vi "Build FilePath By Rule.vi"(8 "error in (no error)":errorcluster, 10 "FileNameRule":T1={"Rule"=enum."Fixed File Name", "Path"=path "", "filename"="data.tdms"}) -> (0 "error out":errorcluster, 3 "File":path)   [LabVIEW 2017]
uses:
  _FileName Rule.ctl
  <userlib>/_OpenG.lib/file/file.llb/Append Path to Root if Relative - Scalar__ogtk.vi
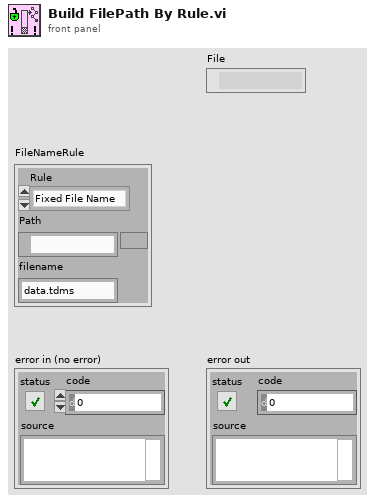
[diagram p1: front panel]
types:
  T1 = typedef "_FileName Rule.ctl" = cluster{"Rule":enum16{"Fixed File Name", "Indexed File Name", "TimeBased File Name"}, "Path":path, "filename":string}
  T2 = enum16{"Fixed File Name", "Indexed File Name", "TimeBased File Name"}
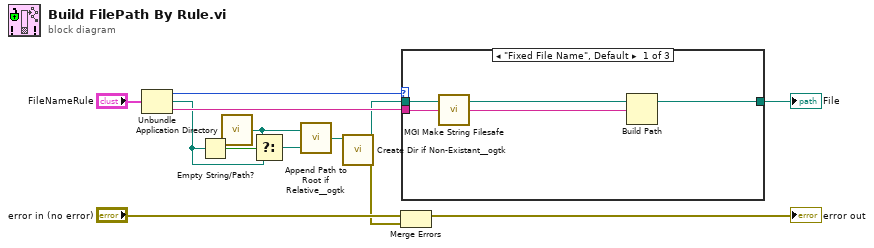
[diagram p0: block diagram]
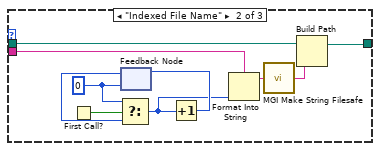
[diagram p2: hidden frame]
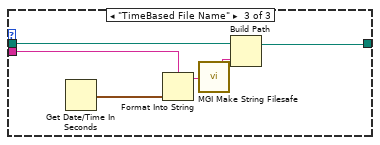
[diagram p3: hidden frame]
diagram:
  n1 = Unbundle("FileNameRule") -> ("Rule"=w13:T2, "Path"=w8:path, "filename"=w12:string)
  n2 = Empty String/Path?(string/path=w8) -> (empty?=w9:bool)
  n3 = call <vilib>:"Application Directory.vi"() -> ("Application Directory"=w3:path)
  n4 = Select(t=w3, s=w9, f=w8) -> (s? t:f=w2:path)
  n5 = call-poly <userlib>:"Append Path to Root if Relative__ogtk.vi"("Absolute or Relative Path"=w2, "Root Path"=w3) -> ("Absolute or Appended Path"=w1:path)
  n6 = call <userlib>:"Create Dir if Non-Existant__ogtk.vi"("Directory Path"=w1) -> ("error out"=w4:errorcluster, "dup Directory Path"=w11:path)  [unwired: 8 in, 1 out]
  n7 = Merge Errors("error in (no error)", w4) -> (→"error out":errorcluster)
  n8 = case shown="\"Fixed File Name\", Default" w13 {
    tunnel: w11 -> [w17 w25 w32]
    tunnel: w12 -> [w16 w27 w33]
    tunnel: [w15 w24 w31] -> w7
    frame "Fixed File Name", Default {
      n9 = call <userlib>:"MGI Make String Filesafe.vi"("String In"=w16) -> ("Filesafe String Out"=w14:string)
      n10 = Build Path(base path=w17, name or relative path=w14) -> (appended path=w15:path)
    }
    frame "Indexed File Name" {
      w19 = 0 ("t")
      n11 = First Call?() -> (First Call?: T/F=w22:bool)
      n12 = feedback #1(w19) -> (w21:i32)
      n13 = Select(t=w19, s=w22, f=w21) -> (s? t:f=w18:i32)
      n14 = Increment(x=w18) -> (x+1=w20:i32)
      n15 = feedback-in #1(w20) -> ()
      n16 = Format Into String(format string=w27, w18) -> (resulting string=w26:string)  [unwired: 2 in, 1 out]
      n17 = call <userlib>:"MGI Make String Filesafe.vi"("String In"=w26) -> ("Filesafe String Out"=w23:string)
      n18 = Build Path(base path=w25, name or relative path=w23) -> (appended path=w24:path)
    }
    frame "TimeBased File Name" {
      n19 = Get Date/Time In Seconds() -> (seconds since 1Jan1904=w30:timestamp)
      n20 = Format Into String(format string=w33, w30) -> (resulting string=w29:string)  [unwired: 2 in, 1 out]
      n21 = call <userlib>:"MGI Make String Filesafe.vi"("String In"=w29) -> ("Filesafe String Out"=w28:string)
      n22 = Build Path(base path=w32, name or relative path=w28) -> (appended path=w31:path)
    }
  }
  "File" <- w7
